vi "Flow Tags.vi"(11 "Flow Module Configs":T1[](array[typedef])) -> (1 "Flow Tags":T5, 2 "Flow Module Tags Array":T5[](array[typedef]), 3 "All  Numeric Tags 4":string[](array[string]), 4 "All Boolean Tags 4":string[](array[string]))   [LabVIEW 2018]
uses:
  Bronkhorst M14 Flow Meter/Tag Cluster.ctl
  Flow Module Folder/Feed Module/Controls/Flow Module Config Cluster.ctl
  <vilib>/Utility/miscctls.llb/LVPoint32TypeDef.ctl
  Flow Module Folder/Feed Module/Controls/Flow Module Settings Cluster.ctl
  Mettler Toledo/Controls/Settings Cluster.ctl
  Flow Module Folder/Flow Module.lvlib
  Mettler Toledo/Mettler Toledo.lvlib
panel:
  # "Flow Meter Settings"
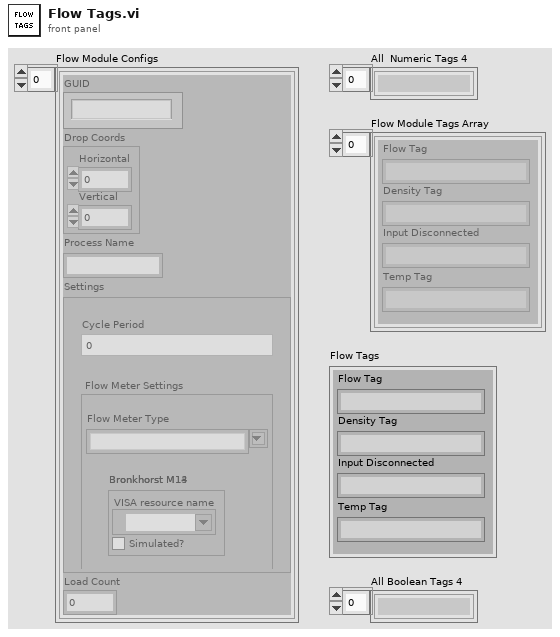
[diagram p1: front panel]
types:
  T1 = typedef "Flow Module.lvlib/Flow Module Config Cluster.ctl" = cluster{"GUID":string, "Drop Coords":T2, "Process Name":string, "Settings":T3, "Load Count":i32}
  T2 = typedef "LVPoint32TypeDef.ctl" = cluster{"Horizontal":i32, "Vertical":i32}
  T3 = typedef "Flow Module.lvlib/Flow Module Settings Cluster.ctl" = cluster{"Cycle Period":dbl, "Bronkhorst M13":T4, "Flow Meter Type":string, "Bronkhorst M14":T4}
  T4 = typedef "Mettler Toledo.lvlib/Settings Cluster.ctl" = cluster{"VISA resource name":refnum<visa-resource-name>, "Simulated?":bool}
  T5 = typedef "Flow Module.lvlib/Tag Cluster.ctl" = cluster{"Flow Tag":string, "Input Disconnected":string, "Density Tag":string, "Temp Tag":string}
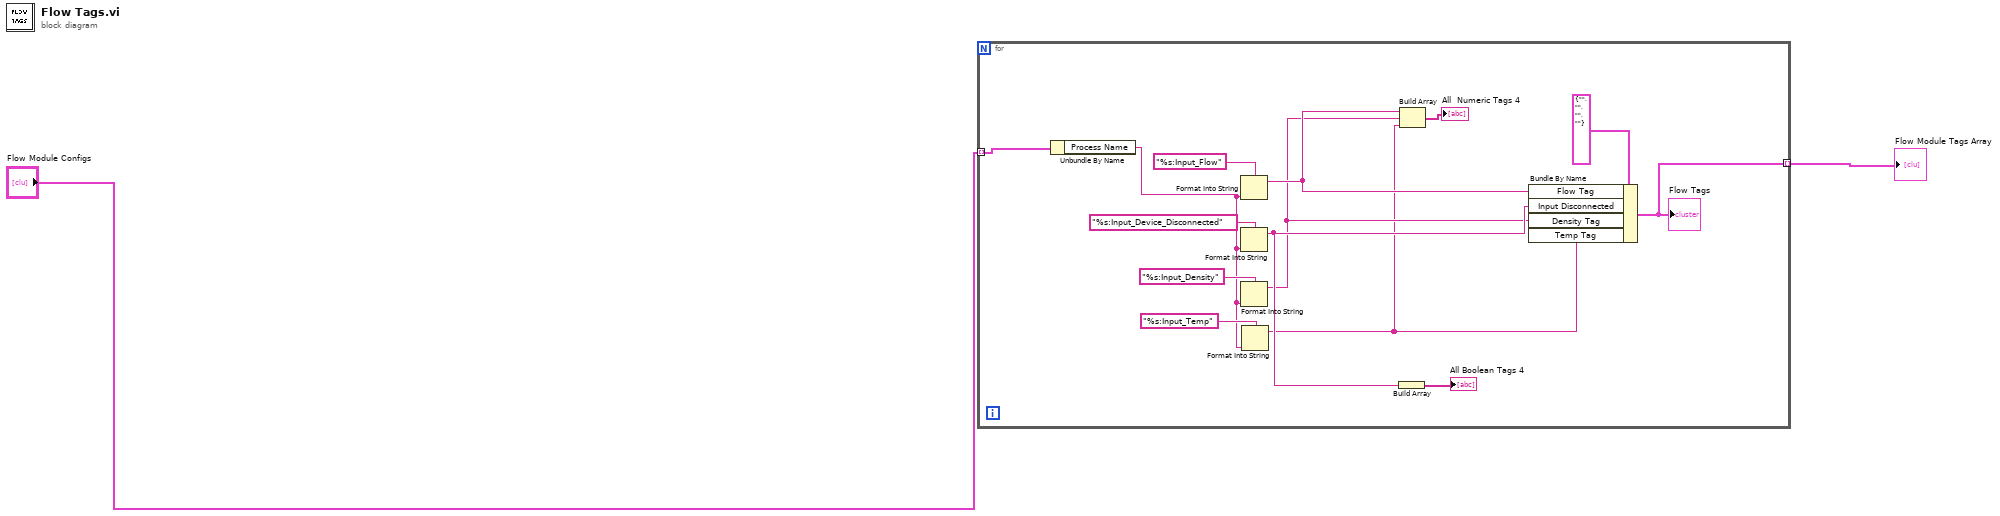
[diagram p0: block diagram]
diagram:
  n1 = for {
    tunnel: "Flow Module Configs" -> [w4] mode=indexing
    tunnel: [w3] -> w2 mode=indexing
    n2 = Unbundle By Name(w4) -> ("Process Name"=w5:string)
    n3 = Format Into String(format string="%s:Input_Flow", w5) -> (resulting string=w12:string)  [unwired: 2 in, 1 out]
    n4 = Format Into String(format string="%s:Input_Device_Disconnected", w5) -> (resulting string=w11:string)  [unwired: 2 in, 1 out]
    n5 = Format Into String(format string="%s:Input_Density", w5) -> (resulting string=w9:string)  [unwired: 2 in, 1 out]
    n6 = Format Into String(format string="%s:Input_Temp", w5) -> (resulting string=w6:string)  [unwired: 2 in, 1 out]
    n7 = Build Array(w11) -> (→"All Boolean Tags 4":string[])
    n8 = Build Array(w12, w9, w6) -> (→"All  Numeric Tags 4":string[])
    n9 = Bundle By Name(cluster=T5 {"Flow Tag"="", "Input Disconnected"="", "Density Tag"="", "Temp Tag"=""} ("Flow Tags 2"), "Flow Tag"=w12, "Input Disconnected"=w11, "Density Tag"=w9, "Temp Tag"=w6) -> (w3:T5)
    "Flow Tags" <- w3
  }
  "Flow Module Tags Array" <- w2
